vi "Get Most Recent Image16.vi"(8 "error in (no error)":errorcluster, 10 "size":u32, 11 "arr":i16[](array[numeric])) -> (0 "error out":errorcluster, 2 "function return":u32, 3 "arr out":i16[](array[numeric]))   [LabVIEW 2018, in "AndorSDK.lvlib"]
doc: "EXPNETTYPE unsigned int WINAPI GetMostRecentImage16(WORD * arr, unsigned long size);"
uses:
  AndorSDK.lvlib
  ATMCD32D.dll
  OwnVIs/AndorOWN.lvlib
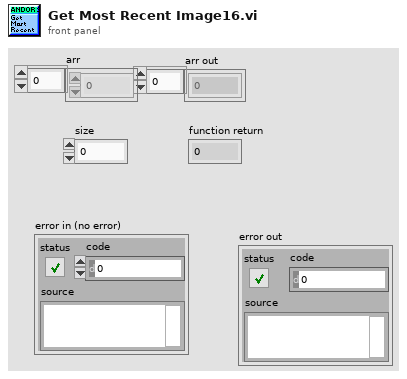
[diagram p1: front panel]
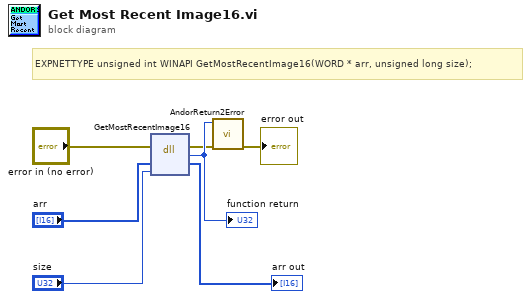
[diagram p0: block diagram]
diagram:
  # "EXPNETTYPE unsigned int WINAPI GetMostRecentImage16(WORD * arr, unsigned long size);"
  n1 = dll-call lib="C:/Users/e14user/Documents/LabVIEW software/GitRepo/lib/ANDOR/Andor SDK/ATMCD32D.*" fn="GetMostRecentImage16"(error in="error in (no error)", "arr"="arr", "size"="size") -> (error out=w1:errorcluster, "return type"=w2:u32, "arr"=→"arr out":i16[])  [unwired: 3 in, 1 out]
  "function return" <- w2
  n2 = call "AndorReturn2Error.vi"("error in (no error)"=w1, "Camera return"=w2) -> ("error out"=→"error out":errorcluster)  [unwired: 9 in]
